vi "spill_param_tcp_server.vi"(6 "tcp_error_in":errorcluster, 7 "port":u16=9999, 8 "spill_id":refnum<vi>, 9 "EOS":refnum<vi>, 10 "BOS":refnum<vi>, 11 "User Event in":refnum<user-event>) -> (3 "server_status":string, 4 "tcp_error_out":errorcluster)   [LabVIEW 2019]
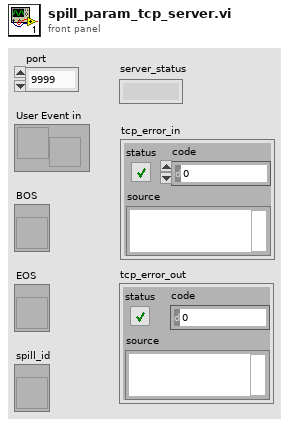
[diagram p1: front panel]
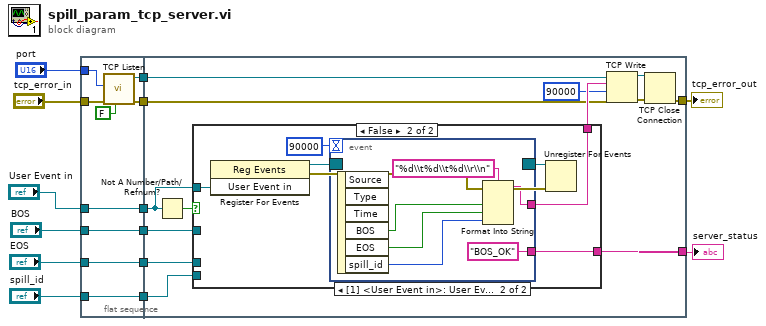
[diagram p0: block diagram]
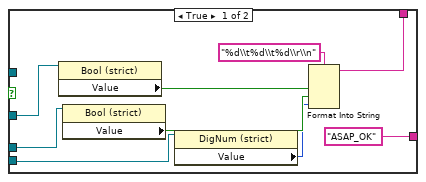
[diagram p2: hidden frame]
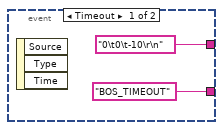
[diagram p3: hidden frame]
diagram:
  n1 = flat-sequence {
    tunnel: "port" -> [w18]
    tunnel: "tcp_error_in" -> [w19]
    tunnel: "User Event in" -> [w20]
    tunnel: "BOS" -> [w21]
    tunnel: "EOS" -> [w22]
    tunnel: "spill_id" -> [w23]
    tunnel: [w23] -> w6
    tunnel: [w22] -> w5
    tunnel: [w21] -> w4
    tunnel: [w20] -> w3
    tunnel: [w16] -> w2
    tunnel: [w15] -> w1
    tunnel: [w33] -> w11
    tunnel: [w29] -> w8
    tunnel: w6 -> [w36]
    tunnel: w5 -> [w35]
    tunnel: w4 -> [w34]
    tunnel: w3 -> [w31]
    tunnel: w2 -> [w25]
    tunnel: w1 -> [w24]
    frame #0 {
      n2 = call <vilib>:"TCP Listen.vi"("resolve remote address (T)"=FALSE, "error in (no error)"=w19, "port"=w18) -> ("error out"=w16:errorcluster, "connection ID"=w15:refnum<k5>)  [unwired: 4 in, 3 out]
    }
    frame #1 {
      n3 = Not A Number/Path/Refnum?(number/path/refnum=w31) -> (NaN/Path/Refnum?=w32:bool)
      n4 = case shown="False" w32 {
        tunnel: [w42 w51] -> w30
        tunnel: w31 -> [_ w47]
        tunnel: ["ASAP_OK" w46] -> w33
        tunnel: w34 -> [w40 _]
        tunnel: w35 -> [w38 _]
        tunnel: w36 -> [w37 _]
        frame True {
          n5 = property on="Property Node" class="Bool (strict)"(reference=w40) -> ("Value"=w39:bool)  [unwired: 1 in, 2 out]
          n6 = property on="Property Node" class="Bool (strict)"(reference=w38) -> ("Value"=w44:bool)  [unwired: 1 in, 2 out]
          n7 = property on="Property Node" class="DigNum (strict)"(reference=w37) -> ("Value"=w43:i32)  [unwired: 1 in, 2 out]
          n8 = Format Into String(format string="%d\\t%d\\t%d\\r\\n", w39, w44, w43) -> (resulting string=w42:string)  [unwired: 2 in, 1 out]
        }
        frame False {
          n9 = register-events(w47) -> (reference out=w50:refnum<event-registration>, error out=w48:errorcluster)  [unwired: 2 in]
          n10 = event shown="[1] <User Event in>: User Event" {
            selector: w50 -> [_ _]
            dyn-events: [_ _] -> w49
            timeout: 90000 -> [_ _]
            tunnel: ["0\t0\t-10\r\n" w60] -> w51
            tunnel: ["BOS_TIMEOUT" "BOS_OK"] -> w46
            event Timeout {
              n11 = event-data() -> ()  [unwired: 1 in, 3 out]
            }
            event User Event {
              n12 = event-data() -> ("BOS"=w57:bool, "EOS"=w56:bool, "spill_id"=w55:i32)  [unwired: 1 in, 3 out]
              n13 = Format Into String(format string="%d\\t%d\\t%d\\r\\n", w57, w56, w55) -> (resulting string=w60:string)  [unwired: 2 in, 1 out]
            }
          }
          n14 = Unregister For Events(event registration refnum=w49, error in=w48) -> ()  [unwired: 1 out]
        }
      }
      n15 = TCP Write(connection ID=w24, data in=w30, error in (no error)=w25, 9:90000 ("timeout ms (25000)")) -> (connection ID out=w27:refnum<k5>, error out=w26:errorcluster)  [unwired: 1 out]
      n16 = TCP Close Connection(connection ID=w27, error in (no error)=w26) -> (error out=w29:errorcluster)  [unwired: 1 in, 1 out]
    }
  }
  "server_status" <- w11
  "tcp_error_out" <- w8
